vi "9_VI_Storage_Status.vi"(8 "error in":errorcluster, 11 "File Path Control":path=path "u:/") -> (0 "File storage error out":errorcluster={"status"=TRUE, "code"=1430, "source"="Get Volume Info in 9_VI_Storage_Status.vi<APPEND>\n/"}, 3 "Storage Status":string="  0 GB capacity with0.000000 MB free (NaN%)")   [LabVIEW 2019]
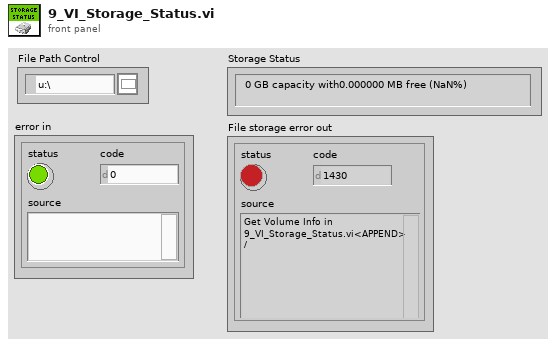
[diagram p1: front panel]
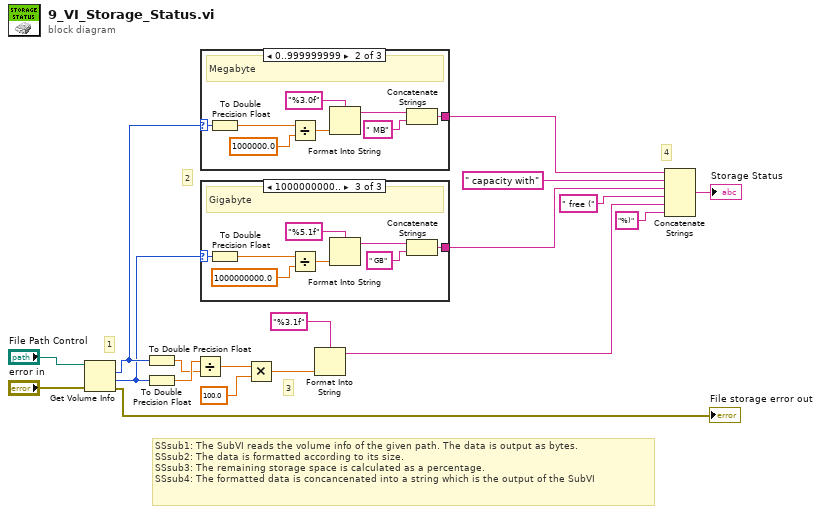
[diagram p0: block diagram]
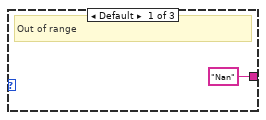
[diagram p2: hidden frame]
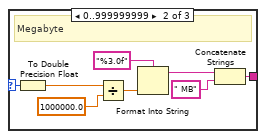
[diagram p3: hidden frame]
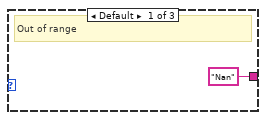
[diagram p4: hidden frame]
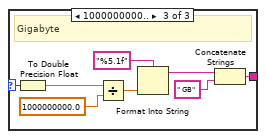
[diagram p5: hidden frame]
diagram:
  # "SSsub1: The SubVI reads the volume info of the given path. The data is output as bytes.\nSSsub2: The data is formatted according to its size.\nSSsub3: The remaining storage space is calculated as a percentage.\nSSsub4: The formatted data is concancenated into a string which is the output of the SubVI"
  # "3"
  # "4"
  # "2"
  # "1"
  n1 = Get Volume Info(8:"error in", 11:"File Path Control") -> (0:→"File storage error out":errorcluster, 1:w3:i64, 2:w6:i64)  [unwired: 3 out]
  n2 = To Double Precision Float(number=w6) -> (double precision float=w7:dbl)
  n3 = To Double Precision Float(number=w3) -> (double precision float=w8:dbl)
  n4 = Divide(x=w8, y=w7) -> (x/y=w9:dbl)
  n5 = case shown="0..999999999" w6 {
    selector: w6 -> [_ w20 w31]
    tunnel: ["Nan" w21 w30] -> w4
    frame Default {
      # "Out of range"
    }
    frame 0..999999999 {
      # "Megabyte"
      n6 = To Double Precision Float(number=w20) -> (double precision float=w26:dbl)
      n7 = Divide(x=w26, y=1000000.0) -> (x/y=w23:dbl)
      n8 = Format Into String(format string="%3.0f", w23) -> (resulting string=w25:string)  [unwired: 2 in, 1 out]
      n9 = Concatenate Strings(w25, " MB" ("string")) -> (w21:string)
    }
    frame 1000000000.. {
      # "Gigabyte"
      n10 = To Double Precision Float(number=w31) -> (double precision float=w34:dbl)
      n11 = Divide(x=w34, y=1000000000.0) -> (x/y=w29:dbl)
      n12 = Format Into String(format string="%5.1f", w29) -> (resulting string=w33:string)  [unwired: 2 in, 1 out]
      n13 = Concatenate Strings(w33, " GB" ("string")) -> (w30:string)
    }
  }
  n14 = case shown="1000000000.." w3 {
    selector: w3 -> [_ w37 w48]
    tunnel: ["Nan" w38 w47] -> w2
    frame Default {
      # "Out of range"
    }
    frame 0..999999999 {
      # "Megabyte"
      n15 = To Double Precision Float(number=w37) -> (double precision float=w43:dbl)
      n16 = Divide(x=w43, y=1000000.0) -> (x/y=w40:dbl)
      n17 = Format Into String(format string="%3.0f", w40) -> (resulting string=w42:string)  [unwired: 2 in, 1 out]
      n18 = Concatenate Strings(w42, " MB" ("string")) -> (w38:string)
    }
    frame 1000000000.. {
      # "Gigabyte"
      n19 = To Double Precision Float(number=w48) -> (double precision float=w51:dbl)
      n20 = Divide(x=w51, y=1000000000.0) -> (x/y=w46:dbl)
      n21 = Format Into String(format string="%5.1f", w46) -> (resulting string=w50:string)  [unwired: 2 in, 1 out]
      n22 = Concatenate Strings(w50, " GB" ("string")) -> (w47:string)
    }
  }
  n23 = Multiply(x=w9, y=100.0) -> (x*y=w12:dbl)
  n24 = Format Into String(format string="%3.1f", w12) -> (resulting string=w13:string)  [unwired: 2 in, 1 out]
  n25 = Concatenate Strings(w4, " capacity with" ("string"), w2, " free (" ("string"), w13, "%)" ("string")) -> (→"Storage Status":string)
